vi "Initialize.vi"(4 "MainProgQEvent":refnum<user-event>, 5 "BaseDataPath":path, 6 "MainProgQ":refnum<queue>, 7 "Experiment Path":path, 8 "ErrIn (NoErr)":errorcluster caption="entrée d'erreur (pas d'erreur)", 9 "Session":string, 10 "SubPanel Refs":refnum<vi>[](array[refnum]), 11 "Experiment In":refnum<class "Experiment.lvclass"> caption="DNL_LabVIEW Object in") -> (0 "error out":errorcluster caption="sortie d'erreur", 2 "PanScanFunc":string[](array[string]), 3 "Experiment Out":refnum<class "Experiment.lvclass"> caption="DNL_LabVIEW Object out")   [LabVIEW 2019, in "Experiment.lvclass"]
uses:
  Experiment.lvclass
  Experiment.lvclass/Experiment.ctl
  DevicesClass/BaseDevice/BaseDevice.lvclass/BaseDevice.ctl
  DevicesClass/BaseDevice/Accessor/SetBaseDataPath.vi
  DevicesClass/BaseDevice/BaseDevice.lvclass
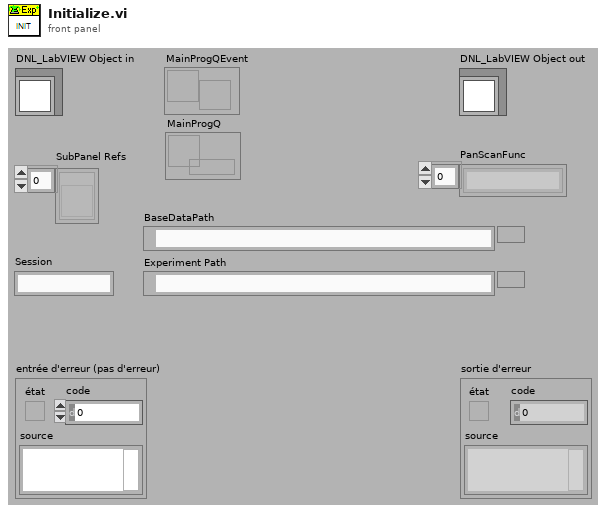
[diagram p1: front panel]
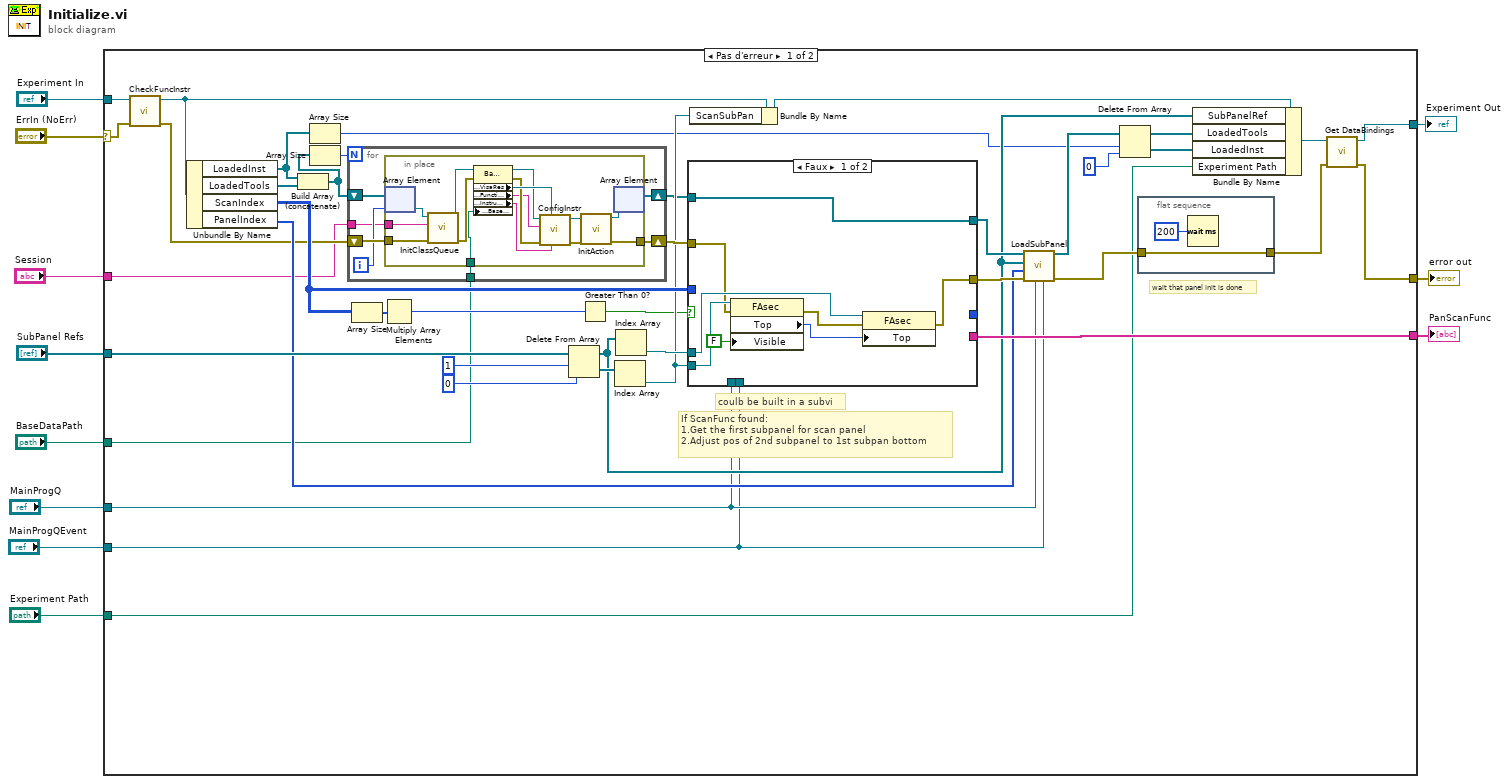
[diagram p0: block diagram]
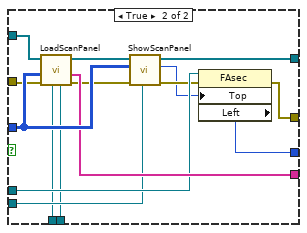
[diagram p2: hidden frame]
diagram:
  n1 = case shown="Pas d'erreur" "ErrIn (NoErr)" {
    selector: "ErrIn (NoErr)" -> [w40 w101]
    tunnel: [w16 w101] -> w10
    tunnel: [w17 w100] -> w8
    tunnel: "Experiment In" -> [w42 w100]
    tunnel: "SubPanel Refs" -> [w50 _]
    tunnel: [w45 _] -> w6
    tunnel: "Session" -> [w30 _]
    tunnel: "MainProgQ" -> [w29 _]
    tunnel: "MainProgQEvent" -> [w28 _]
    tunnel: "Experiment Path" -> [w13 _]
    tunnel: "BaseDataPath" -> [w12 _]
    frame No Error {
      # "wait that panel init is done"
      # "coulb be built in a subvi"
      # "If ScanFunc found:\n1.Get the first subpanel for scan panel\n2.Adjust pos of 2nd subpanel to 1st subpan bottom"
      n2 = call "CheckFuncInstr.vi"("error in (no error)"=w40, "Experiment en entrée"=w42) -> ("error out"=w39:errorcluster, "Experiment en sortie"=w41:refnum<class "Experiment.lvclass">)  [unwired: 8 in]
      n3 = Unbundle By Name(w41) -> ("LoadedInst"=w27:refnum<class "BaseDevice.lvclass">[], "LoadedTools"=w26:refnum<class "BaseDevice.lvclass">[], "ScanIndex"=w49:i32[][], "PanelIndex"=w44:i32[])
      n4 = Build Array (concatenate)(w27, w26) -> (w20:refnum<class "BaseDevice.lvclass">[])
      n5 = Array Size(array=w27) -> (size(s)=w22:i32)
      n6 = Array Size(array=w20) -> (size(s)=w19:i32)
      n7 = for {
        N: w19 -> [_]
        shift-right: [w84] -> w48
        shift-left: w39 -> [w83]
        shift-right: [w80] -> w31
        shift-left: w20 -> [w82]
        tunnel: w30 -> [w79]
        tunnel: w12 -> [w78]
        i -> [w81]
        n8 = in-place {
          in-place-border: [w99] -> w84
          in-place-border: w83 -> [w98]
          in-place-border: w79 -> [w96]
          in-place-border: w78 -> [w86]
          n9 = in-place-array #1(w82, w81) -> (w93:refnum<class "BaseDevice.lvclass">)
          n10 = call "InitClassQueue.vi"("ErrorIn(No Error)"=w98, "Session"=w96, "BaseDevice.lvclass"=w93) -> ("sortie d'erreur"=w91:errorcluster, "BaseDevice.lvclass Out"=w87:refnum<class "BaseDevice.lvclass">)  [unwired: 5 in, 2 out]
          n11 = property class="BaseDevice.lvclass"(reference=w87, error in=w91, "Accessor:BaseDataPath"=w86) -> (reference out=w85:refnum<class "BaseDevice.lvclass">, error out=w90:errorcluster, "Accessor:VisaRes"=w92:refnum<visa-resource-name>, "Accessor:Function"=w89:string, "Accessor:InstrumentName"=w88:string)
          n12 = call-dynamic "ConfigInstr.vi"("InstrumentName"=w88, "VisaRessIn"=w92, "error in (no error)"=w90, "Function"=w89, "Device en entrée"=w85) -> ("error out"=w94:errorcluster, "Device en sortie"=w95:refnum<class "BaseDevice.lvclass">)  [unwired: 5 in]
          n13 = call-dynamic "InitAction.vi"("error in (no error)"=w94, "Device en entrée"=w95) -> ("error out"=w99:errorcluster, "Device en sortie"=w97:refnum<class "BaseDevice.lvclass">)  [unwired: 8 in]
          n14 = in-place-array #1(w97) -> (w80:refnum<class "BaseDevice.lvclass">[])  [unwired: 1 out]
        }
      }
      n15 = Array Size(array=w49) -> (size(s)=w52:i32[])
      n16 = Multiply Array Elements(1:w52) -> (0:w51:i32)
      n17 = Delete From Array(array=w50, length=1 ("longueur"), index=0 ("indice")) -> (deleted portion=w36:refnum<vi>[], array with subset deleted=w32:refnum<vi>[])
      n18 = Greater Than 0?(x=w51) -> (x > 0?=w33:bool)
      n19 = Index Array(array=w36) -> (element=w34:refnum<vi>)  [unwired: 1 in]
      n20 = Index Array(array=w32) -> (element=w35:refnum<vi>)  [unwired: 1 in]
      n21 = case shown="Faux" w33 {
        tunnel: w49 -> [_ w77]
        tunnel: w48 -> [w57 w76]
        tunnel: w31 -> [w62 w75]
        tunnel: [w55 w74] -> w47
        tunnel: [w62 w73] -> w46
        tunnel: [_ w72] -> w45
        tunnel: w35 -> [w59 w69]
        tunnel: w34 -> [w61 w66]
        tunnel: w29 -> [_ w65]
        tunnel: w28 -> [_ w64]
        tunnel: [_ w63] -> _
        frame False {
          n22 = property class="FAsec"(reference=w61, error in=w57, "Visible"=FALSE) -> (error out=w56:errorcluster, "Top"=w58:i32)  [unwired: 1 out]
          n23 = property class="FAsec"(reference=w59, error in=w56, "Top"=w58) -> (error out=w55:errorcluster)  [unwired: 1 out]
        }
        frame True {
          n24 = call "LoadScanPanel.vi"("MainProgQEvent"=w64, "MainProgQ"=w65, "error in (no error)"=w76, "ScanIndex"=w77, "LoadedInst"=w75) -> ("sortie d'erreur"=w71:errorcluster, "PanScanFunc"=w72:string[], "LoadedInst Out"=w70:refnum<class "BaseDevice.lvclass">[])  [unwired: 3 in, 1 out]
          n25 = call "ShowScanPanel.vi"("SubPanel"=w66, "error in (no error)"=w71, "ScanIndex"=w77, "LoadedInst"=w70) -> ("sortie d'erreur"=w68:errorcluster, "NextPanPos"=w67:u32, "LoadedInst Out"=w73:refnum<class "BaseDevice.lvclass">[])  [unwired: 5 in]
          n26 = property class="FAsec"(reference=w69, error in=w68, "Top"=w67) -> (error out=w74:errorcluster, "Left"=w63:i32)  [unwired: 1 out]
        }
      }
      n27 = Bundle By Name(cluster=w41, "ScanSubPan"=w34) -> (w43:refnum<class "Experiment.lvclass">)
      n28 = call "LoadSubPanel.vi"("MainProgQEvent"=w28, "MainProgQ"=w29, "error in (no error)"=w47, "PanelIndex"=w44, "SubPanel Refs"=w32, "LoadedInst"=w46) -> ("sortie d'erreur"=w15:errorcluster, "LoadedInst Out"=w25:refnum<class "BaseDevice.lvclass">[])  [unwired: 4 in]
      n29 = Delete From Array(array=w25, length=w22, index=0) -> (deleted portion=w23:refnum<class "BaseDevice.lvclass">[], array with subset deleted=w24:refnum<class "BaseDevice.lvclass">[])
      n30 = flat-sequence {
        tunnel: w15 -> [w54]
        tunnel: [w54] -> w14
        frame #0 {
          n31 = Wait (ms)(milliseconds to wait=u32 200 ("attente (ms)")) -> ()  [unwired: 1 out]
        }
      }
      n32 = Bundle By Name(cluster=w43, "SubPanelRef"=w32, "LoadedTools"=w24, "LoadedInst"=w23, "Experiment Path"=w13) -> (w18:refnum<class "Experiment.lvclass">)
      n33 = call "Get DataBindings.vi"("error in"=w14, "Experiment.lvclass"=w18) -> ("error out"=w16:errorcluster, "Experiment.lvclass out"=w17:refnum<class "Experiment.lvclass">)  [unwired: 8 in]
    }
    frame Error {
    }
  }
  "error out" <- w10
  "Experiment Out" <- w8
  "PanScanFunc" <- w6
